vi "Configure Detector Characteristics.vi"(6 "Auto Reference Channel (T: Enable)":bool=TRUE, 7 "Auto Offset Detector (T: Enable)":bool=TRUE, 8 "error in (no error)":errorcluster, 9 "Manual Reference Channel (0: Average)":i32(ring) items=["Average", "Peak", "Sample", "Negative Peak", "Normal"], 10 "Manual Offset Detector Type (0: Average)":i32(ring) items=["Average", "Peak", "Sample", "Negative Peak", "Normal"], 11 "VISA resource name":refnum<visa-resource-name>) -> (0 "error out":errorcluster, 3 "VISA resource name out":refnum<visa-resource-name>)   [LabVIEW 2018, in "Agilent MXA Series.lvlib"]
doc: "Configures the detector characteristics under Spectrum Emission Mask measurement type."
uses:
  Agilent MXA Series.lvlib
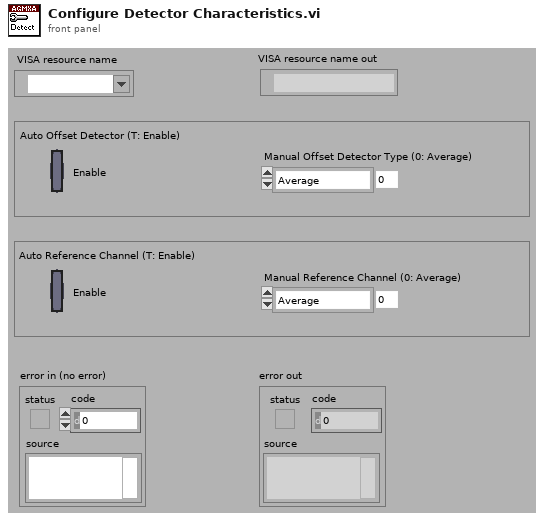
[diagram p1: front panel]
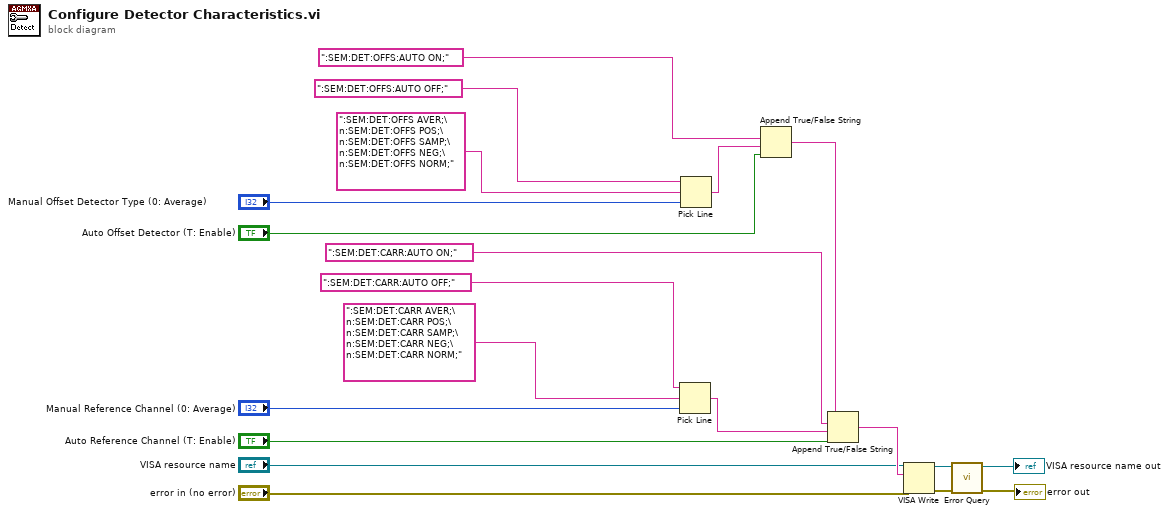
[diagram p0: block diagram]
diagram:
  n1 = Pick Line(string ("")=":SEM:DET:CARR:AUTO OFF;", multi-line string=":SEM:DET:CARR AVER;\n:SEM:DET:CARR POS;\n:SEM:DET:CARR SAMP;\n:SEM:DET:CARR NEG;\n:SEM:DET:CARR NORM;", line index="Manual Reference Channel (0: Average)") -> (output string=w10:string)
  n2 = Pick Line(string ("")=":SEM:DET:OFFS:AUTO OFF;", multi-line string=":SEM:DET:OFFS AVER;\n:SEM:DET:OFFS POS;\n:SEM:DET:OFFS SAMP;\n:SEM:DET:OFFS NEG;\n:SEM:DET:OFFS NORM;", line index="Manual Offset Detector Type (0: Average)") -> (output string=w16:string)
  n3 = Append True/False String(1:"Auto Offset Detector (T: Enable)", 2:w16, 3:":SEM:DET:OFFS:AUTO ON;") -> (0:w8:string)  [unwired: 1 in]
  n4 = Append True/False String(1:"Auto Reference Channel (T: Enable)", 2:w10, 3:":SEM:DET:CARR:AUTO ON;", 4:w8) -> (0:w7:string)
  n5 = VISA Write(VISA resource name="VISA resource name", write buffer=w7, error in (no error)="error in (no error)") -> (VISA resource name out=w4:refnum<visa-resource-name>, error out=w3:errorcluster)  [unwired: 1 out]
  n6 = call "Error Query.vi"("error in (no error)"=w3, "VISA resource name"=w4) -> ("error out"=→"error out":errorcluster, "VISA resource name out"=→"VISA resource name out":refnum<visa-resource-name>)  [unwired: 6 in, 2 out]
